vi "Arduino_LDR.vi"() -> ()   [LabVIEW 2024]
uses:
  <vilib>/Instr/_visa.llb/VISA Configure Serial Port (Instr).vi
panel:
  out "LED1":bool
  out "LED2":bool
  out "light intensity":dbl(slide) scale=0.0..500.0
  in  "stop":bool
  in  "VISA resource name":refnum<visa-resource-name>
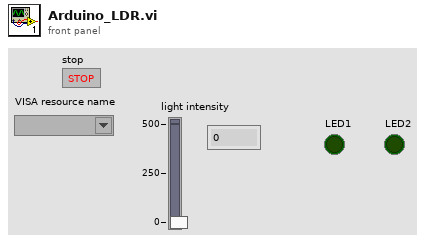
[diagram p1: front panel]
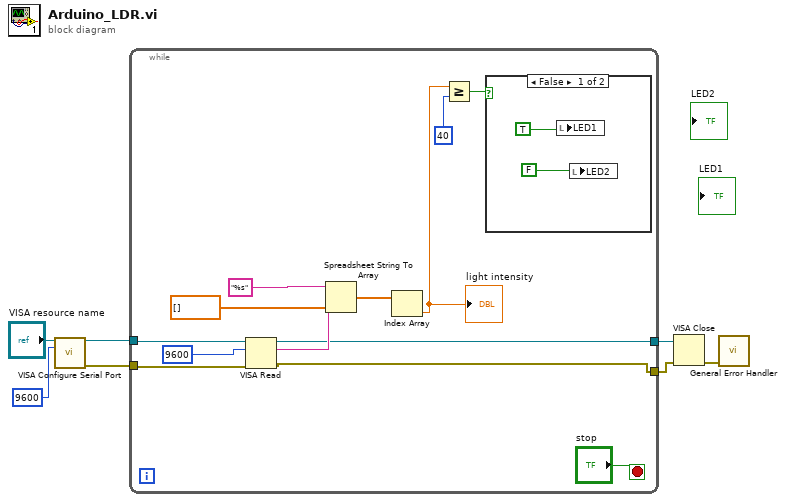
[diagram p0: block diagram]
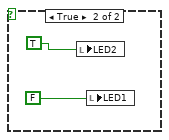
[diagram p2: hidden frame]
diagram:
  n1 = call-poly "VISA Configure Serial Port"("VISA resource name"="VISA resource name", "baud rate (9600)"=9600) -> ("VISA resource name out"=w5:refnum<visa-resource-name>, "error out"=w4:errorcluster)  [unwired: 12 in]
  n2 = while {
    tunnel: w5 -> [w20]
    tunnel: w4 -> [w19]
    tunnel: [w10] -> w3
    tunnel: [w9] -> w2
    stop <- "stop" stop-if-true
    n3 = VISA Read(VISA resource name=w20, byte count=9600, error in (no error)=w19) -> (VISA resource name out=w10:refnum<visa-resource-name>, read buffer=w17:string, error out=w9:errorcluster)  [unwired: 1 out]
    n4 = Spreadsheet String To Array(format string="%s", spreadsheet string=w17, array type (2D Dbl)=dbl[] []) -> (array=w14:dbl[])  [unwired: 1 in]
    n5 = Index Array(array=w14) -> (element=w8:dbl)  [unwired: 1 in]
    "light intensity" <- w8
    n6 = Greater Or Equal?(x=w8, y=40) -> (x >= y?=w11:bool)
    n7 = case shown="False" w11 {
      frame False {
        n8 = local write "LED1"(TRUE) -> ()
        n9 = local write "LED2"(FALSE) -> ()
      }
      frame True {
        n10 = local write "LED2"(TRUE) -> ()
        n11 = local write "LED1"(FALSE) -> ()
      }
    }
  }
  n12 = VISA Close(VISA resource name=w3, error in (no error)=w2) -> (error out=w1:errorcluster)
  n13 = call <vilib>:"General Error Handler.vi"("error in (no error)"=w1) -> ()  [unwired: 10 in, 5 out]
